vi "Szimulacio2.vi"() -> ()   [LabVIEW 2013]
uses:
  Parameterek.ctl
  Bemeno_Parameterek.ctl
  Szamolt_Parameterek.ctl
panel:
  in  "Tab Control":T1(tab)
  out "Számolt paraméterek":T2
  in  "Bemeneti paraméterek":T3={"rho PCM"=1100.0, "rho kulso"=28.3, "Dkulso"=0.1, "nkulso"=10, "rho kozepso"=28.3, "Dkozepso"=0.06, "nkozepso"=6, "rho belso"=28.3, "Dbelso"=0.1, "nbelso"=10, "Alfa kulso"=0.015, "Alfa belso"=0.006, "Alfa kont"=0.03, "lambda_kulso"=5.0000000000105516e-05, "lambda_kozepso"=5e-05, "lambda_belso"=5e-05, "hpcm_olv"=140.0, "Top_also"=24.0, "Top_felso"=28.0, "ckulso"=1.13, "ckozepso"=1.13, "cbelso"=1.13, "cpcm_szilard"=1.9, "lambda_pcm"=0.00018, "Vlevego"=0.446, "rho levego"=1.3, "clevego"=1.0, "cpcm_olvnelkul"=0.0, "cpcm_foly"=1.5, "Xpcm_kulso"=0.3, "Xpcm_belso"=0.3}
  in  "OK Button 2":bool
  in  "Belso levegõ\n kiindulási hõmérséklet [°C]":dbl=20.5
  in  "stop":bool
  in  "OK Button":bool
  in  "t_sim [nap]":dbl=14.0 caption="Szimuláció ideje [nap]"
  in  "mód":enum16{"szinusz", "ugrás"}(ring)=enum."ugrás"
  in  "T_kulso_0":dbl=20.5 caption="Kiindulási hõmérsékletek [°C]" format="%#_13g"
  in  "Parameterek":T4={"rholevego"=0.0, "Vlevego"=0.0, "Mlevego"=0.0, "clevego"=0.0, "rho PCM"=1100.0, "rho kulso"=28.3, "Dkulso"=0.1, "nkulso"=10, "dkulso"=0.0, "vkulso"=0.0, "rho kozepso"=28.3, "Dkozepso"=0.06, "nkozepso"=6, "dkozepso"=0.0, "vkozepso"=0.0, "mkozepso"=0.0, "mkulso"=0.0, "rho belso"=28.3, "Dbelso"=0.1, "nbelso"=10, "dbelso"=0.0, "vbelso"=0.0, "mbelso"=0.0, "Xpcm_kulso"=0.3, "Xpcm_belso"=0.3, "mpcm_kulso"=0.0, "mpcm_belso"=0.0, "mkulso_pcm"=0.0, "mbelso_pcm"=0.0, "ckulso"=1.13, "ckozepso"=1.13, "cbelso"=1.13, "cpcm_szilard"=1.9, "cpcm_foly"=1.5, "ckulso_Topalatt"=0.0, "cbelso_Topalatt"=0.0, "ckulso_Topfelett"=0.0, "cbelso_Topfelett"=0.0, "hpcm_olv"=140.0, "ckulso_eff_Tolv"=0.0, "cbelso_eff_Tolv"=0.0, "Qkulso_op_also"=0.0, "Qkulso_op_felso"=0.0, "Qbelso_op_also"=0.0, "Qbelso_op_felso"=0.0, "lambda_kulso"=5e-05, "lambda_kozepso"=5e-05, "lambda_belso"=5e-05, "lambda_pcm"=0.00018, "VXpcm_kulso"=0.0, "VXpcm_belso"=0.0, "lambda_kulsoPCM"=0.0, "lambda_belsoPCM"=0.0, "Alfa_kulso"=0.015, "Alfa_belso"=0.006, "Alfa_kont"=0.03, "Top_also"=24.0, "Top_felso"=28.0, "cpcm_olvnelkul"=0.0, "Tbelsolevego_0"=22.0}
  in  "T_max  [°C]":dbl=33.5
  in  "T_min [°C]":dbl=20.5
  out "T_kulsolevego":dbl[](graph)
  out "T_kozepso":dbl[][](graph) caption="Középsõ rétegek hõmérséklete"
  out "T_kulso":dbl[][](graph) caption="Külsõ PCM rétegek hõmérséklete"
  out "T_belso":dbl[][](graph) caption="Belsõ PCM rétegek hõmérséklete"
  out "T_belsolevego":dbl[](graph) caption="Belsõ levegõ hõmérséklete"
  out "Hõáram a külsõ PCM rétegen belül":dbl[][](graph)
  out "Hõáram a középsõ rétegen belül":dbl[][](graph)
  out "Hõáram a belsõ rétegen belül":dbl[][](graph)
  out "F bel_in":dbl[](graph) caption="Hõáram a a belsõ falon befelé"
  out "F kozbel":dbl[](graph) caption="Hõáram a középsõ és belsõ réteg között"
  out "F kulkoz":dbl[](graph) caption="Hõáram a külsõ és középsõ réteg között"
  out "Hõáram  a falon befelé":dbl[](graph)
  out "Q_belsolevego":dbl[](graph) caption="Belsõ levegõ hõtartalma"
  out "Q_kozepso":dbl[][](graph) caption="Középsõ rétegek hõtartalma"
  out "Q_kulso":dbl[][](graph) caption="Külsõ PCM rétegek hõtartalma"
  out "Q_belso":dbl[][](graph) caption="Belsõ PCM rétegek hõtartalma"
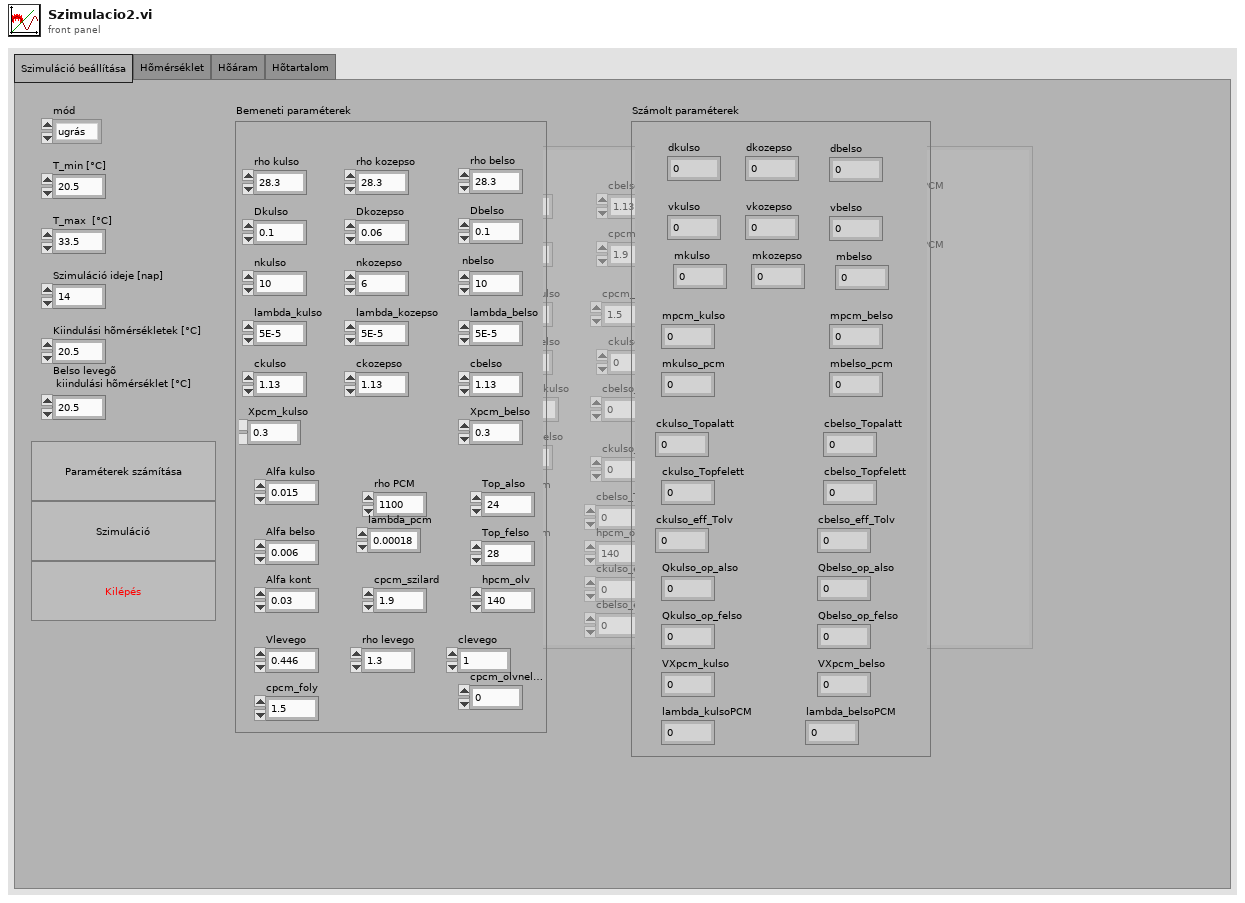
[diagram p1: front panel]
types:
  T1 = enum32{"Szimuláció beállítása", "Hõmérséklet", "Hõáram", "Hõtartalom"}
  T2 = typedef "Szamolt_Parameterek.ctl" = cluster{"dkulso":dbl, "dkozepso":dbl, "dbelso":dbl, "vkulso":dbl, "vkozepso":dbl, "vbelso":dbl, "mkulso":dbl, "mkozepso":dbl, "mbelso":dbl, "mpcm_kulso":dbl, "mpcm_belso":dbl, "mkulso_pcm":dbl, "mbelso_pcm":dbl, "ckulso_Topalatt":dbl, "ckulso_Topfelett":dbl, "cbelso_Topalatt":dbl, "cbelso_Topfelett":dbl, "ckulso_eff_Tolv":dbl, "cbelso_eff_Tolv":dbl, "Qkulso_op_also":dbl, "Qkulso_op_felso":dbl, "Qbelso_op_also":dbl, "Qbelso_op_felso":dbl, "VXpcm_kulso":dbl, "VXpcm_belso":dbl, "lambda_kulsoPCM":dbl, "lambda_belsoPCM":dbl}
  T3 = typedef "Bemeno_Parameterek.ctl" = cluster{"rho PCM":dbl, "rho kulso":dbl, "Dkulso":dbl, "nkulso":i32, "rho kozepso":dbl, "Dkozepso":dbl, "nkozepso":i32, "rho belso":dbl, "Dbelso":dbl, "nbelso":i32, "Alfa kulso":dbl, "Alfa belso":dbl, "Alfa kont":dbl, "lambda_kulso":dbl, "lambda_kozepso":dbl, "lambda_belso":dbl, "hpcm_olv":dbl, "Top_also":dbl, "Top_felso":dbl, "ckulso":dbl, "ckozepso":dbl, "cbelso":dbl, "cpcm_szilard":dbl, "lambda_pcm":dbl, "Vlevego":dbl, "rho levego":dbl, "clevego":dbl, "cpcm_olvnelkul":dbl, "cpcm_foly":dbl, "Xpcm_kulso":dbl, "Xpcm_belso":dbl}
  T4 = typedef "Parameterek.ctl" = cluster{"rholevego":dbl, "Vlevego":dbl, "Mlevego":dbl, "clevego":dbl, "rho PCM":dbl, "rho kulso":dbl, "Dkulso":dbl, "nkulso":i32, "dkulso":dbl, "vkulso":dbl, "rho kozepso":dbl, "Dkozepso":dbl, "nkozepso":i32, "dkozepso":dbl, "vkozepso":dbl, "mkozepso":dbl, "mkulso":dbl, "rho belso":dbl, "Dbelso":dbl, "nbelso":i32, "dbelso":dbl, "vbelso":dbl, "mbelso":dbl, "Xpcm_kulso":dbl, "Xpcm_belso":dbl, "mpcm_kulso":dbl, "mpcm_belso":dbl, "mkulso_pcm":dbl, "mbelso_pcm":dbl, "ckulso":dbl, "ckozepso":dbl, "cbelso":dbl, "cpcm_szilard":dbl, "cpcm_foly":dbl, "ckulso_Topalatt":dbl, "cbelso_Topalatt":dbl, "ckulso_Topfelett":dbl, "cbelso_Topfelett":dbl, "hpcm_olv":dbl, "ckulso_eff_Tolv":dbl, "cbelso_eff_Tolv":dbl, "Qkulso_op_also":dbl, "Qkulso_op_felso":dbl, "Qbelso_op_also":dbl, "Qbelso_op_felso":dbl, "lambda_kulso":dbl, "lambda_kozepso":dbl, "lambda_belso":dbl, "lambda_pcm":dbl, "VXpcm_kulso":dbl, "VXpcm_belso":dbl, "lambda_kulsoPCM":dbl, "lambda_belsoPCM":dbl, "Alfa_kulso":dbl, "Alfa_belso":dbl, "Alfa_kont":dbl, "Top_also":dbl, "Top_felso":dbl, "cpcm_olvnelkul":dbl, "Tbelsolevego_0":dbl}
  T5 = cluster{"Q_belsolevego":dbl[], "T_kulso_levego_vektor":dbl[], "Hõaram a falon be":dbl[], "F_bel_in":dbl[], "F_kulso_vektor":dbl[][], "T_belsolevego":dbl[], "Q_kulso_aktualis_vektor":dbl[][], "T belso vektor":dbl[][], "T kulso vektor":dbl[][], "Q_belso_aktualis_vektor":dbl[][], "F_kulkoz":dbl[], "F_kozepso_vektor":dbl[][], "Q_kozepso_aktualis_vektor":dbl[][], "T kozepso vektor":dbl[][], "F_kozbel":dbl[], "F_belso_vektor":dbl[][]}
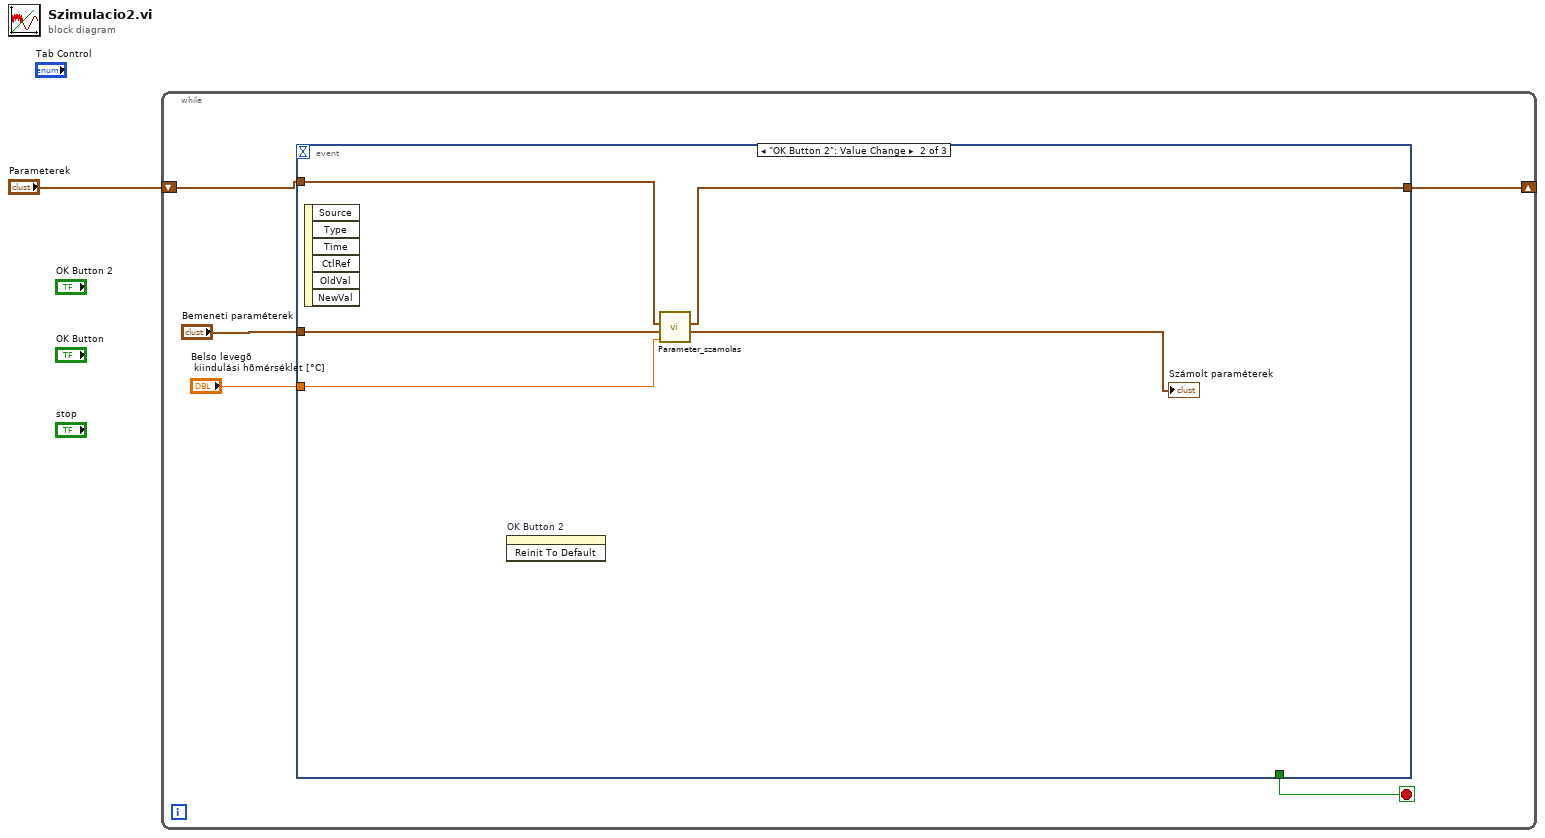
[diagram p0: block diagram]
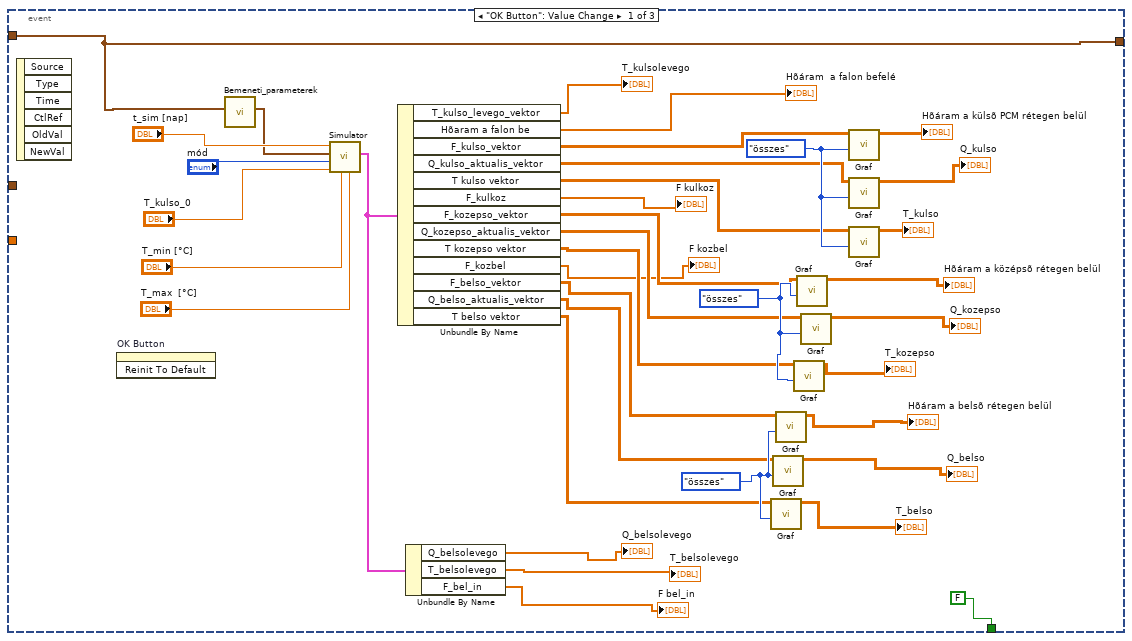
[diagram p2: hidden frame]
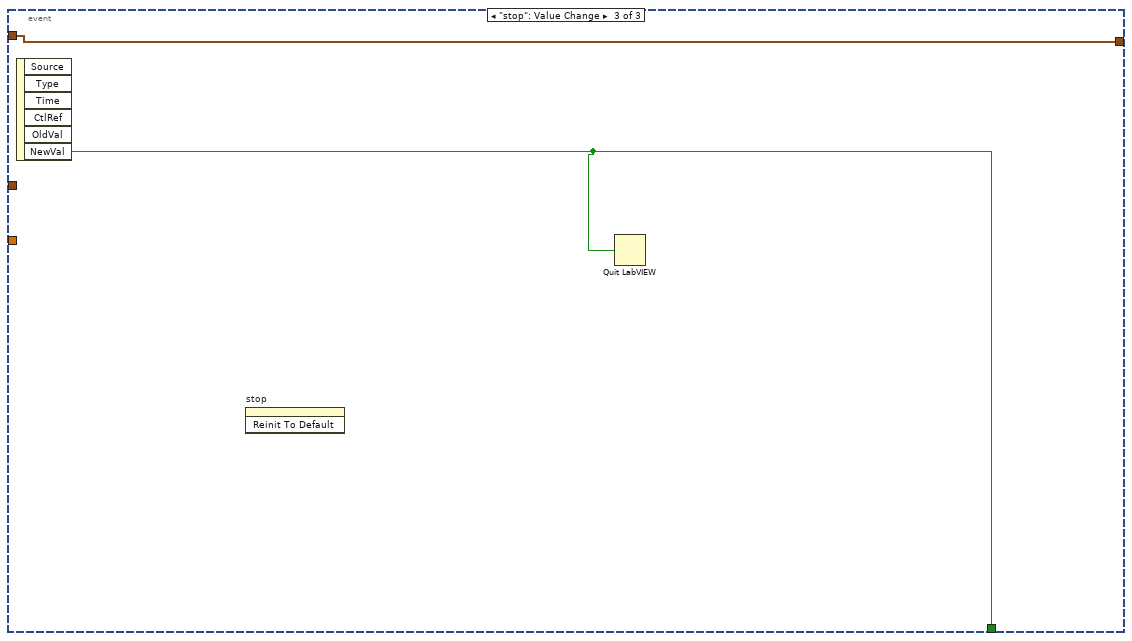
[diagram p3: hidden frame]
diagram:
  n1 = while {
    shift-right: [w4] -> _
    shift-left: "Parameterek" -> [w5]
    stop <- w6 stop-if-true
    n2 = event shown="[1] \"OK Button 2\": Value Change" {
      selector: _ -> [_ _ _]
      dyn-events: _ -> [_ _ _]
      timeout: _ -> [_ _ _]
      tunnel: [FALSE _ w50] -> w6
      tunnel: w5 -> [w20 w48 w49]
      tunnel: "Bemeneti paraméterek" -> [_ w46 _]
      tunnel: [w20 w47 w49] -> w4
      tunnel: "Belso levegõ\n kiindulási hõmérséklet [°C]" -> [_ w45 _]
      event "OK Button": Value Change {
        w35 = enum16{"három", "összes", "eleje", "vége"}."összes" ("mód")
        w36 = enum16{"három", "összes", "eleje", "vége"}."összes" ("mód")
        w39 = enum16{"három", "összes", "eleje", "vége"}."összes" ("mód")
        n3 = event-data() -> ()  [unwired: 1 in, 6 out]
        n4 = invoke on="OK Button" class="Bool" method="Reinit To Default"() -> ()  [unwired: 3 in, 3 out]
        n5 = call "Bemeneti_parameterek.vi"("Parameterek"=w20) -> ("Parameterek 2"=w41:T4)  [unwired: 10 in]
        n6 = call "Simulator.vi"("T_max"="T_max  [°C]", "T_min"="T_min [°C]", "Q_kulso_0"="T_kulso_0", "mód"="mód", "Parameterek in"=w41, "t_sim [nap]"="t_sim [nap]") -> ("output cluster"=w23:T5)  [unwired: 5 in]
        n7 = Unbundle By Name(w23) -> ("T_kulso_levego_vektor"=→"T_kulsolevego":dbl[], "Hõaram a falon be"=→"Hõáram  a falon befelé":dbl[], "F_kulso_vektor"=w32:dbl[][], "Q_kulso_aktualis_vektor"=w31:dbl[][], "T kulso vektor"=w30:dbl[][], "F_kulkoz"=→"F kulkoz":dbl[], "F_kozepso_vektor"=w29:dbl[][], "Q_kozepso_aktualis_vektor"=w28:dbl[][], "T kozepso vektor"=w27:dbl[][], "F_kozbel"=→"F kozbel":dbl[], "F_belso_vektor"=w26:dbl[][], "Q_belso_aktualis_vektor"=w25:dbl[][], "T belso vektor"=w24:dbl[][])
        n8 = Unbundle By Name(w23) -> ("Q_belsolevego"=→"Q_belsolevego":dbl[], "T_belsolevego"=→"T_belsolevego":dbl[], "F_bel_in"=→"F bel_in":dbl[])
        n9 = call "Graf.vi"("mód"=w35, "F_kulso_vektor"=w24) -> ("Grafikonra"=→"T_belso":dbl[][])  [unwired: 9 in]
        n10 = call "Graf.vi"("mód"=w35, "F_kulso_vektor"=w25) -> ("Grafikonra"=→"Q_belso":dbl[][])  [unwired: 9 in]
        n11 = call "Graf.vi"("mód"=w35, "F_kulso_vektor"=w26) -> ("Grafikonra"=→"Hõáram a belsõ rétegen belül":dbl[][])  [unwired: 9 in]
        n12 = call "Graf.vi"("mód"=w36, "F_kulso_vektor"=w27) -> ("Grafikonra"=→"T_kozepso":dbl[][])  [unwired: 9 in]
        n13 = call "Graf.vi"("mód"=w36, "F_kulso_vektor"=w29) -> ("Grafikonra"=→"Hõáram a középsõ rétegen belül":dbl[][])  [unwired: 9 in]
        n14 = call "Graf.vi"("mód"=w36, "F_kulso_vektor"=w28) -> ("Grafikonra"=→"Q_kozepso":dbl[][])  [unwired: 9 in]
        n15 = call "Graf.vi"("mód"=w39, "F_kulso_vektor"=w32) -> ("Grafikonra"=→"Hõáram a külsõ PCM rétegen belül":dbl[][])  [unwired: 9 in]
        n16 = call "Graf.vi"("mód"=w39, "F_kulso_vektor"=w31) -> ("Grafikonra"=→"Q_kulso":dbl[][])  [unwired: 9 in]
        n17 = call "Graf.vi"("mód"=w39, "F_kulso_vektor"=w30) -> ("Grafikonra"=→"T_kulso":dbl[][])  [unwired: 9 in]
      }
      event "OK Button 2": Value Change {
        n18 = event-data() -> ()  [unwired: 1 in, 6 out]
        n19 = invoke on="OK Button 2" class="Bool" method="Reinit To Default"() -> ()  [unwired: 3 in, 3 out]
        n20 = call "Parameter_szamolas.vi"("Tbelsolevego_0"=w45, "Bemeneti paraméterek"=w46, "Parameterek"=w48) -> ("Számolt paraméterek"=→"Számolt paraméterek":T2, "Parameterek 2"=w47:T4)  [unwired: 7 in]
      }
      event "stop": Value Change {
        n21 = event-data() -> ("NewVal"=w50:bool)  [unwired: 1 in, 5 out]
        n22 = invoke on="stop" class="Bool" method="Reinit To Default"() -> ()  [unwired: 3 in, 3 out]
        n23 = Quit LabVIEW(quit? (T)=w50) -> ()
      }
    }
  }
